vi "FPGA_AIOpen.vi"(8 "error in (no error)":errorcluster) -> (0 "error out":errorcluster, 3 "AI Reference out":T1)   [LabVIEW 2017]
uses:
  <vilib>/Rock Robotics/SystemInterfaces/AI/FPGA_AIDevRef.ctl
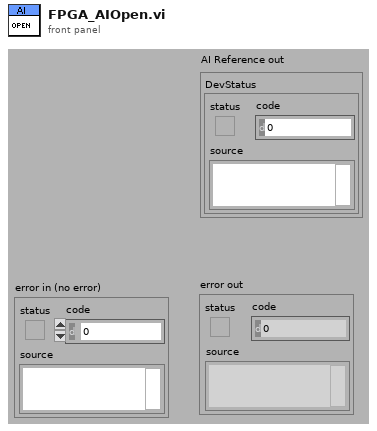
[diagram p1: front panel]
types:
  T1 = typedef "FPGA_AIDevRef.ctl" = cluster{"DevStatus":errorcluster}
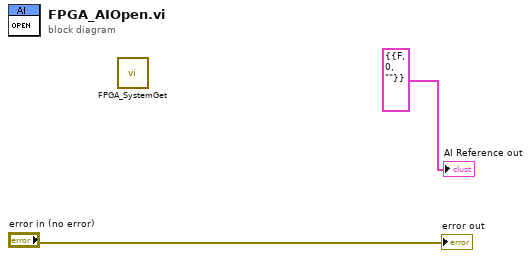
[diagram p0: block diagram]
diagram:
  n1 = call <vilib>:"FPGA_SystemGet.vi"() -> ()  [unwired: 2 in, 10 out]
  "AI Reference out" <- T1 {"DevStatus"={"status"=FALSE, "code"=0, "source"=""}} ("AI Reference out 2")
  "error out" <- "error in (no error)"
